vi "HV SubModule.vi"(8 "Error in":errorcluster, 11 "External Event":refnum<user-event>) -> (0 "Error out":errorcluster)   [LabVIEW 2018, in "HV QMH.lvlib"]
uses:
  HV QMH.lvlib
  CORE/QMH/QMH CORE.lvlib
  CORE/Queue Messaging/Queue Messaging.lvlib
  CORE/Event Messaging/Event Messaging.lvlib
  Configuration/Configuration.lvlib
  Type Defs/Data--cluster.ctl
  CORE/Event Messaging/Type Defs/Event Message--cluster.ctl
types:
  T1 = typedef "HV QMH.lvlib/Data--cluster.ctl" = cluster{"Channels":string[], "Data Array":string[], "Single Data":string, "Single Channel":string}
  T2 = typedef "QMH CORE.lvlib/EventsAndQueues--cluster.ctl" = cluster{"Internal Queue":refnum<queue>, "Internal Event":refnum<user-event>, "External Event":refnum<user-event>}
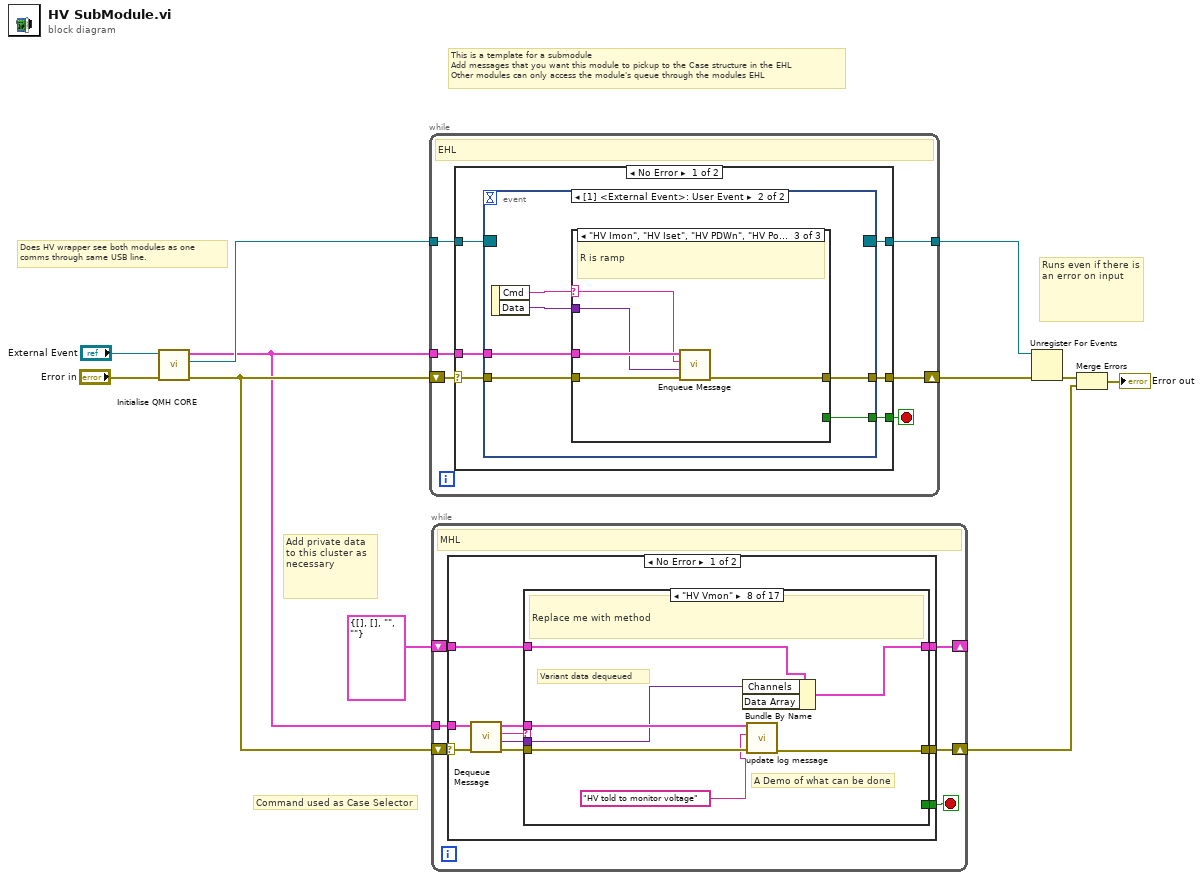
[diagram p0: block diagram]
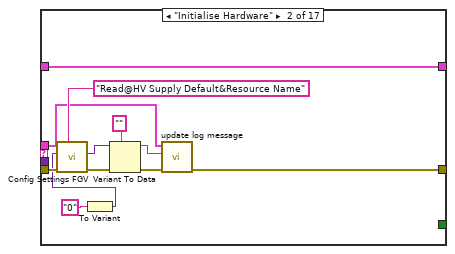
[diagram p3: hidden frame]
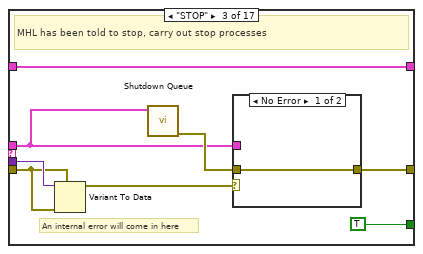
[diagram p4: hidden frame]
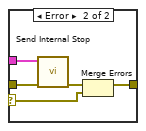
[diagram p5: hidden frame]
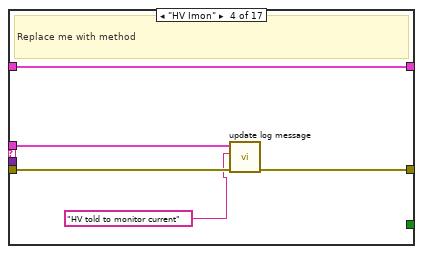
[diagram p6: hidden frame]
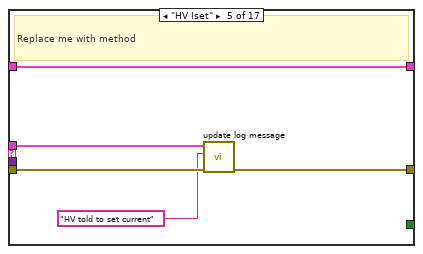
[diagram p7: hidden frame]
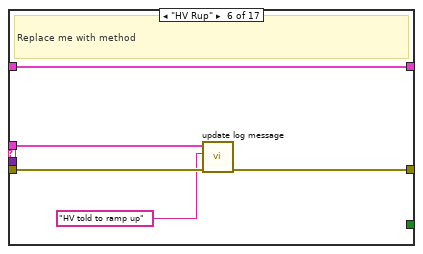
[diagram p8: hidden frame]
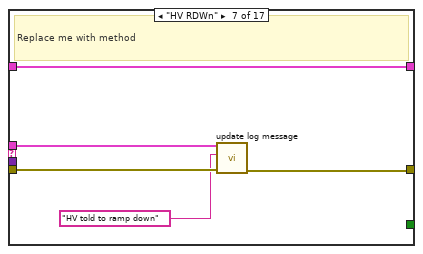
[diagram p9: hidden frame]
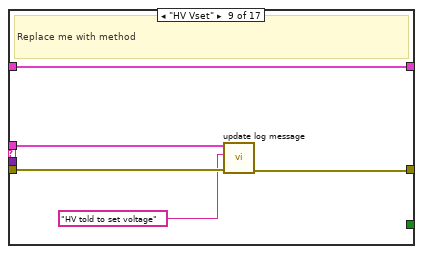
[diagram p10: hidden frame]
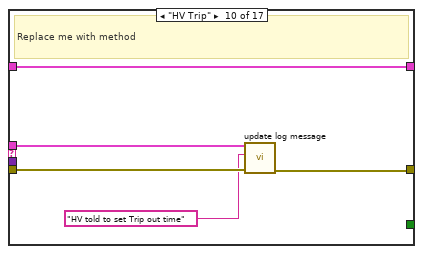
[diagram p11: hidden frame]
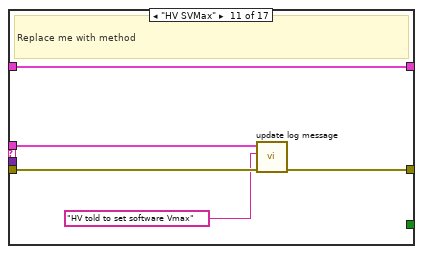
[diagram p12: hidden frame]
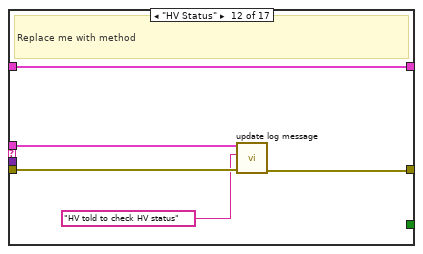
[diagram p13: hidden frame]
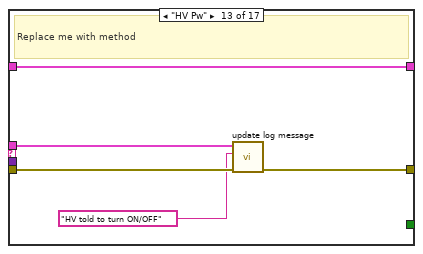
[diagram p14: hidden frame]
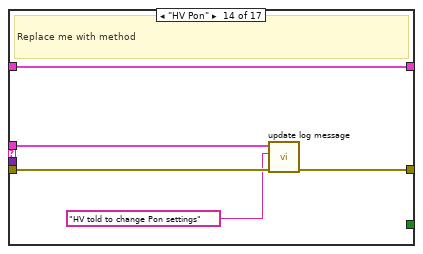
[diagram p15: hidden frame]
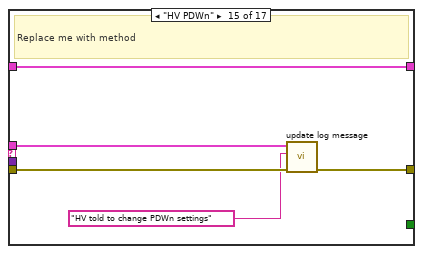
[diagram p16: hidden frame]
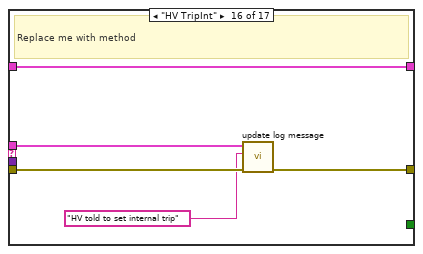
[diagram p17: hidden frame]
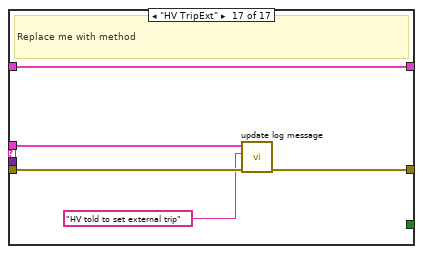
[diagram p18: hidden frame]
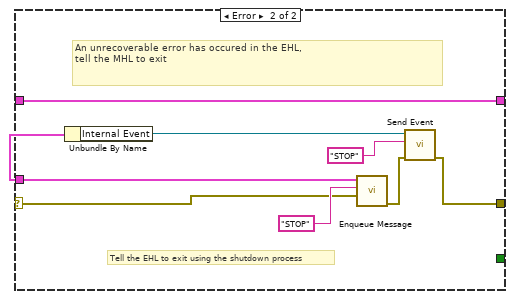
[diagram p19: hidden frame]
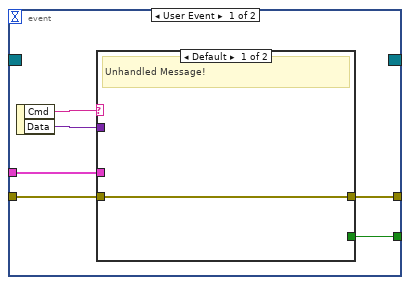
[diagram p20: hidden frame]
diagram:
  # "Command used as Case Selector"
  # "Does HV wrapper see both modules as one\ncomms through same USB line."
  # "Add private data to this cluster as necessary"
  # "This is a template for a submodule\nAdd messages that you want this module to pickup to the Case structure in the EHL\nOther modules can only access the module's queue through the modules EHL"
  # "Runs even if there is an error on input"
  n1 = call "Initialise QMH CORE.vi"("Error in"="Error in", "External Event"="External Event") -> ("Error out"=w11:errorcluster, "Event Registration Refnum"=w10:refnum<event-registration>, "Queue Data"=w1:T2)  [unwired: 7 in]
  n2 = while {
    shift-right: [w15] -> w9
    shift-left: w11 -> [w17]
    tunnel: w1 -> [w16]
    tunnel: w10 -> [w13]
    tunnel: [w12] -> w8
    stop <- w14 stop-if-true
    # "EHL"
    n3 = case shown="No Error" w17 {
      selector: w17 -> [w23 w53]
      tunnel: w16 -> [w22 w54]
      tunnel: [w21 w50] -> w15
      tunnel: [w20 TRUE] -> w14
      tunnel: w13 -> [w19 w51]
      tunnel: [w18 w51] -> w12
      frame No Error {
        n4 = event shown="[1] <External Event>: User Event" {
          selector: w19 -> [_ _]
          dyn-events: [_ _] -> w18
          timeout: _ -> [_ _]
          tunnel: w23 -> [w29 w36]
          tunnel: w22 -> [w25 w33]
          tunnel: [w28 w35] -> w21
          tunnel: [w24 w34] -> w20
          event User Event {
            n5 = event-data() -> ("Cmd"=w27:string, "Data"=w26:variant)  [unwired: 1 in]
            n6 = case shown="Default" w27 {
              tunnel: w29 -> [w30 w31]
              tunnel: [w30 w31] -> w28
              tunnel: w26 -> [_ _]
              tunnel: w25 -> [_ _]
              tunnel: [_ TRUE] -> w24
              frame Default {
                # "Unhandled Message!"
              }
              frame "STOP" {
                # "Internal STOP received, MHL has told EHL to stop"
              }
            }
          }
          event User Event {
            n7 = event-data() -> ("Cmd"=w38:string, "Data"=w37:variant)  [unwired: 1 in]
            n8 = case shown="\"HV Imon\", \"HV Iset\", \"HV PDWn\", \"HV Pon\", \"HV Pw\", \"HV RDWn\", \"HV Rup\", \"HV SVMax\", \"HV Status\", \"HV Trip\", \"HV TripExt\", \"HV TripInt\", \"HV Vmon\", \"HV Vset\", \"Initialise Hardware\"" w38 {
              selector: w38 -> [_ _ w45]
              tunnel: w36 -> [w39 w42 w48]
              tunnel: [w39 w41 w46] -> w35
              tunnel: [_ TRUE _] -> w34
              tunnel: w37 -> [_ _ w44]
              tunnel: w33 -> [_ w40 w47]
              frame Default {
                # "Unhandled Message!"
              }
              frame "STOP" {
                # "External STOP received, Another module has told this one to stop, stop the MHL"
                n9 = call "Enqueue Stop Message.vi"("Error in"=w42, "Queue Data"=w40) -> ("Error out"=w41:errorcluster)  [unwired: 9 in]
              }
              frame "HV Imon", "HV Iset", "HV PDWn", "HV Pon", "HV Pw", "HV RDWn", "HV Rup", "HV SVMax", "HV Status", "HV Trip", "HV TripExt", "HV TripInt", "HV Vmon", "HV Vset", "Initialise Hardware" {
                # "R is ramp"
                n10 = call "Enqueue Message.vi"("Error in"=w48, "Data"=w44, "Cmd"=w45, "Queue Data"=w47) -> ("Error out"=w46:errorcluster)  [unwired: 7 in]
              }
            }
          }
        }
      }
      frame Error {
        # "EHL has generated an unrecoverable error!\nStop the MHL and pass out error"
        n11 = call "Enqueue Stop Message.vi"("Queue Data"=w54) -> ("Error out"=w49:errorcluster)  [unwired: 10 in]
        n12 = Merge Errors(w49, w53) -> (w50:errorcluster)
      }
    }
  }
  n13 = while {
    shift-right: [w58] -> w4
    shift-left: w11 -> [w60]
    tunnel: w1 -> [w59]
    shift-right: [w56] -> _
    shift-left: T1 {"Channels"=[], "Data Array"=[], "Single Data"="", "Single Channel"=""} -> [w55]
    stop <- w57 stop-if-true
    # "MHL"
    n14 = case shown="No Error" w60 {
      selector: w60 -> [w70 w174]
      tunnel: w59 -> [w69 w176]
      tunnel: [w65 w172] -> w58
      tunnel: [w64 _] -> w57
      tunnel: [w62 w171] -> w56
      tunnel: w55 -> [w61 w171]
      frame No Error {
        n15 = call "Dequeue Message.vi"("Error in"=w70, "Queue Data in"=w69) -> ("Error out"=w67:errorcluster, "Data"=w66:variant, "Cmd"=w68:string, "Queue Data out"=w63:T2)  [unwired: 6 in]
        n16 = case shown="\"HV Vmon\"" w68 {
          tunnel: w67 -> [w72 w82 w90 w102 w107 w112 w117 w125 w129 w134 w139 w144 w149 w154 w159 w164 w169]
          tunnel: w66 -> [_ _ w91 _ _ _ _ w121 _ _ _ _ _ _ _ _ _]
          tunnel: [w72 w76 w87 w101 w106 w111 w116 w124 w128 w133 w138 w143 w148 w153 w158 w162 w168] -> w65
          tunnel: [_ _ TRUE _ _ _ _ _ _ _ _ _ _ _ _ _ _] -> w64
          tunnel: w63 -> [_ w75 w86 w100 w105 w110 w115 w123 w127 w132 w137 w142 w147 w152 w157 w163 w167]
          tunnel: [w71 w84 w85 w103 w108 w113 w118 w119 w130 w135 w140 w145 w150 w155 w160 w165 w170] -> w62
          tunnel: w61 -> [w71 w84 w85 w103 w108 w113 w118 w120 w130 w135 w140 w145 w150 w155 w160 w165 w170]
          frame Default {
            # "Unhandled Message!"
          }
          frame "Initialise Hardware" {
            n17 = To Variant(anything="0") -> (Variant=w74:variant)
            n18 = call "Config Settings FGV.vi"("Command"="Read@HV Supply Default&Resource Name", "error in (no error)"=w82, "Data in"=w74) -> ("error out"=w81:errorcluster, "Data out"=w80:variant)  [unwired: 7 in]
            n19 = Variant To Data(error in=w81, type="", Variant=w80) -> (data=w78:string, error out=w79:errorcluster)
            n20 = call "update log message.vi"("error in (no error)"=w79, "Message"=w78, "Queue Data in"=w75) -> ("error out"=w76:errorcluster)  [unwired: 7 in, 1 out]
          }
          frame "STOP" {
            # "An internal error will come in here"
            # "MHL has been told to stop, carry out stop processes"
            n21 = Variant To Data(error in=w90, type=w90, Variant=w91) -> (data=w89:errorcluster)  [unwired: 1 out]
            n22 = call "Shutdown Queue.vi"("Queue Data"=w86) -> ("Error out"=w88:errorcluster)  [unwired: 10 in]
            n23 = case shown="No Error" w89 {
              selector: w89 -> [_ w94]
              tunnel: w88 -> [w93 w98]
              tunnel: [w93 w96] -> w87
              tunnel: w86 -> [_ w97]
              frame No Error {
              }
              frame Error {
                n24 = call "Send Internal Stop.vi"("Error in"=w98, "Queue Data"=w97) -> ("Error out"=w95:errorcluster)  [unwired: 9 in]
                n25 = Merge Errors(w95, w94) -> (w96:errorcluster)
              }
            }
          }
          frame "HV Imon" {
            # "Replace me with method"
            n26 = call "update log message.vi"("error in (no error)"=w102, "Message"="HV told to monitor current", "Queue Data in"=w100) -> ("error out"=w101:errorcluster)  [unwired: 7 in, 1 out]
          }
          frame "HV Iset" {
            # "Replace me with method"
            n27 = call "update log message.vi"("error in (no error)"=w107, "Message"="HV told to set current", "Queue Data in"=w105) -> ("error out"=w106:errorcluster)  [unwired: 7 in, 1 out]
          }
          frame "HV Rup" {
            # "Replace me with method"
            n28 = call "update log message.vi"("error in (no error)"=w112, "Message"="HV told to ramp up", "Queue Data in"=w110) -> ("error out"=w111:errorcluster)  [unwired: 7 in, 1 out]
          }
          frame "HV RDWn" {
            # "Replace me with method"
            n29 = call "update log message.vi"("error in (no error)"=w117, "Message"="HV told to ramp down", "Queue Data in"=w115) -> ("error out"=w116:errorcluster)  [unwired: 7 in, 1 out]
          }
          frame "HV Vmon" {
            # "A Demo of what can be done"
            # "Variant data dequeued"
            # "Replace me with method"
            n30 = Bundle By Name(cluster=w120, "Channels"=w121) -> (w119:T1)  [unwired: 1 in]
            n31 = call "update log message.vi"("error in (no error)"=w125, "Message"="HV told to monitor voltage", "Queue Data in"=w123) -> ("error out"=w124:errorcluster)  [unwired: 7 in, 1 out]
          }
          frame "HV Vset" {
            # "Replace me with method"
            n32 = call "update log message.vi"("error in (no error)"=w129, "Message"="HV told to set voltage", "Queue Data in"=w127) -> ("error out"=w128:errorcluster)  [unwired: 7 in, 1 out]
          }
          frame "HV Trip" {
            # "Replace me with method"
            n33 = call "update log message.vi"("error in (no error)"=w134, "Message"="HV told to set Trip out time", "Queue Data in"=w132) -> ("error out"=w133:errorcluster)  [unwired: 7 in, 1 out]
          }
          frame "HV SVMax" {
            # "Replace me with method"
            n34 = call "update log message.vi"("error in (no error)"=w139, "Message"="HV told to set software Vmax", "Queue Data in"=w137) -> ("error out"=w138:errorcluster)  [unwired: 7 in, 1 out]
          }
          frame "HV Status" {
            # "Replace me with method"
            n35 = call "update log message.vi"("error in (no error)"=w144, "Message"="HV told to check HV status", "Queue Data in"=w142) -> ("error out"=w143:errorcluster)  [unwired: 7 in, 1 out]
          }
          frame "HV Pw" {
            # "Replace me with method"
            n36 = call "update log message.vi"("error in (no error)"=w149, "Message"="HV told to turn ON/OFF", "Queue Data in"=w147) -> ("error out"=w148:errorcluster)  [unwired: 7 in, 1 out]
          }
          frame "HV Pon" {
            # "Replace me with method"
            n37 = call "update log message.vi"("error in (no error)"=w154, "Message"="HV told to change Pon settings", "Queue Data in"=w152) -> ("error out"=w153:errorcluster)  [unwired: 7 in, 1 out]
          }
          frame "HV PDWn" {
            # "Replace me with method"
            n38 = call "update log message.vi"("error in (no error)"=w159, "Message"="HV told to change PDWn settings", "Queue Data in"=w157) -> ("error out"=w158:errorcluster)  [unwired: 7 in, 1 out]
          }
          frame "HV TripInt" {
            # "Replace me with method"
            n39 = call "update log message.vi"("error in (no error)"=w164, "Message"="HV told to set internal trip", "Queue Data in"=w163) -> ("error out"=w162:errorcluster)  [unwired: 7 in, 1 out]
          }
          frame "HV TripExt" {
            # "Replace me with method"
            n40 = call "update log message.vi"("error in (no error)"=w169, "Message"="HV told to set external trip", "Queue Data in"=w167) -> ("error out"=w168:errorcluster)  [unwired: 7 in, 1 out]
          }
        }
      }
      frame Error {
        # "Tell the EHL to exit using the shutdown process"
        # "An unrecoverable error has occured in the EHL, \ntell the MHL to exit"
        n41 = Unbundle By Name(w176) -> ("Internal Event"=w178:refnum<user-event>)
        n42 = call "Enqueue Message.vi"("Data"=w174, "Cmd"="STOP", "Queue Data"=w176) -> ("Error out"=w173:errorcluster)  [unwired: 8 in]
        n43 = call "Send Event.vi"("Error in"=w173, "Cmd"="STOP", "Event Ref"=w178) -> ("Error out"=w172:errorcluster)  [unwired: 7 in, 1 out]
      }
    }
  }
  n44 = Unregister For Events(event registration refnum=w8, error in=w9) -> (error out=w6:errorcluster)
  n45 = Merge Errors(w6, w4) -> (→"Error out":errorcluster)
